vi "Vision Processing.vi"(8 "error in (no error)":errorcluster, 11 "Image Size":T2=enum."320x240") -> ()   [LabVIEW 2015]
uses:
  <vilib>/Rock Robotics/WPI/Camera/WPI_CameraImageSize.ctl
  OS6 VIs/References/Relevant Data.ctl
  Robot Global Data.vi
  <vilib>/vision/NI_Vision_Development_Module.lvlib
panel:
  out "Relevant Data":T1[](array[typedef])
  out "Distance":dbl
  in  "Goal Width":dbl=20.0
  in  "Center Right":dbl=162.0
  in  "Center Left":dbl=153.0
  in  "Mask Color":i32=1
  out "ms to process":u32
  in  "LED Color":T3={"Hue"={91.12518353230051, 179.40124989546868}, "Sat"={197.32142857142858, 255.0}, "Val"={182.14285714285714, 255.0}} {"Hue" scale=0.0..255.0 scale format="%#_3g"}
  out "Qualified Particles":i32
  in  "Aspect Fudge Factor":dbl=1.0
  in  "Min Score Threshold":i32=75
  out "Masked":T4(plugin-control)
  out "Original Image":T4(plugin-control)
  out "fps":dbl
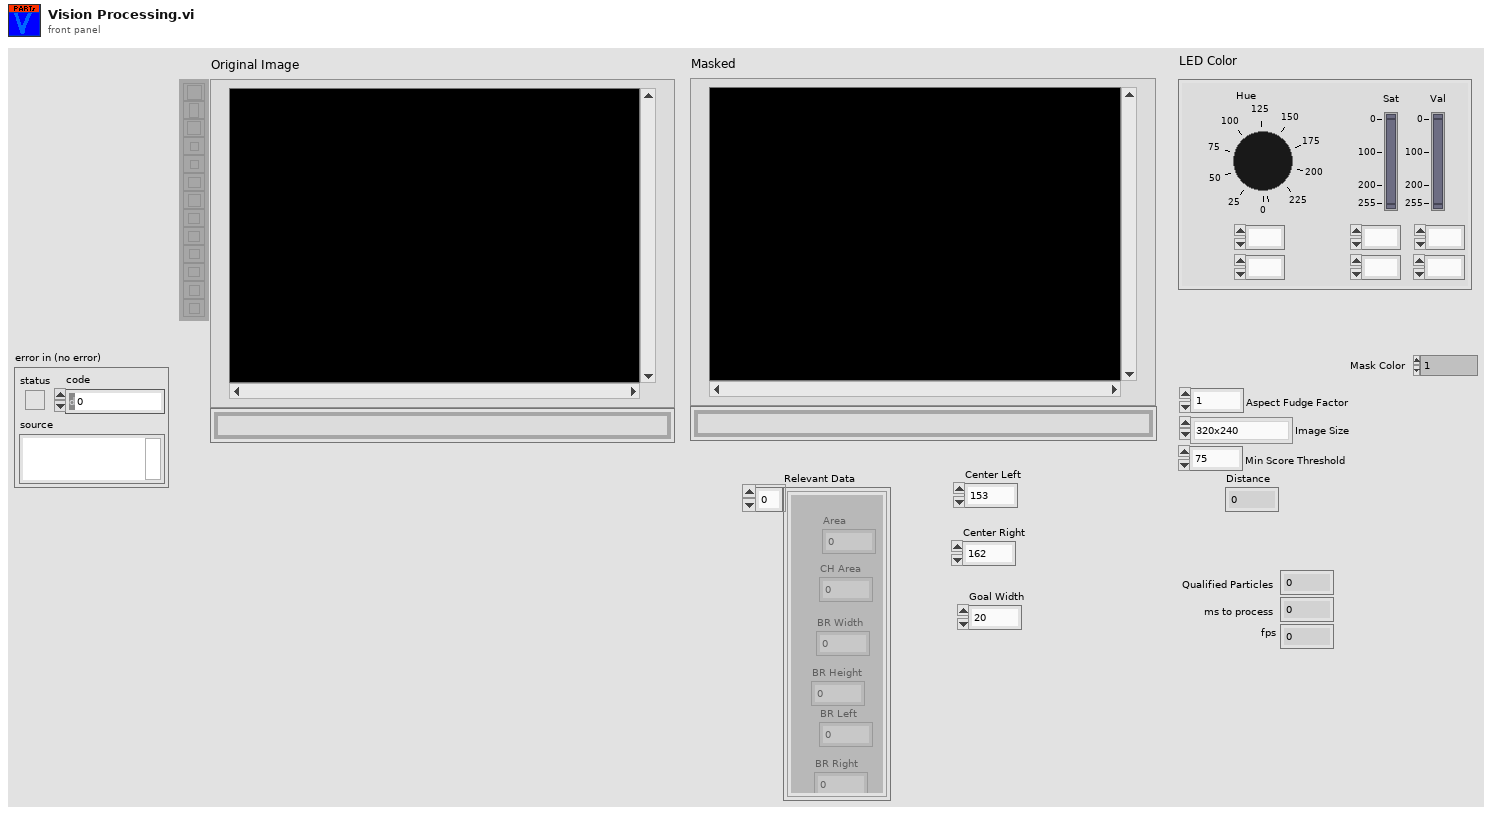
[diagram p1: front panel]
types:
  T1 = typedef "Relevant Data.ctl" = cluster{"Area":dbl, "CH Area":dbl, "BR Width":dbl, "BR Height":dbl, "BR Left":dbl, "BR Right":dbl}
  T2 = typedef "WPI_CameraImageSize.ctl" = enum16{"640x480", "320x240", "160x120", "Custom"}
  T3 = cluster{"Hue":cluster{dbl, dbl}, "Sat":cluster{dbl, dbl}, "Val":cluster{dbl, dbl}}
  T4 = typedef "IMAQ Image.ctl" = refnum<image>
  T5 = typedef "Image Type" = u32
  T6 = typedef "Particle Parameters" = i32
  T7 = typedef "WPI_CameraDevRef.ctl" = cluster{"Camera Address":string, "CameraStatus":errorcluster}
  T8 = cluster{"Goal Left":dbl, "Goal Right":dbl, "Goal Width":dbl}
  T9 = cluster{"Bounding box":cluster{"left":dbl, "top":dbl, "right":dbl, "bottom":dbl}, "Aspect Ratio":dbl, "Area to CH":dbl, "X Mask":dbl, "Y Mask":dbl, "Moment":dbl}[]
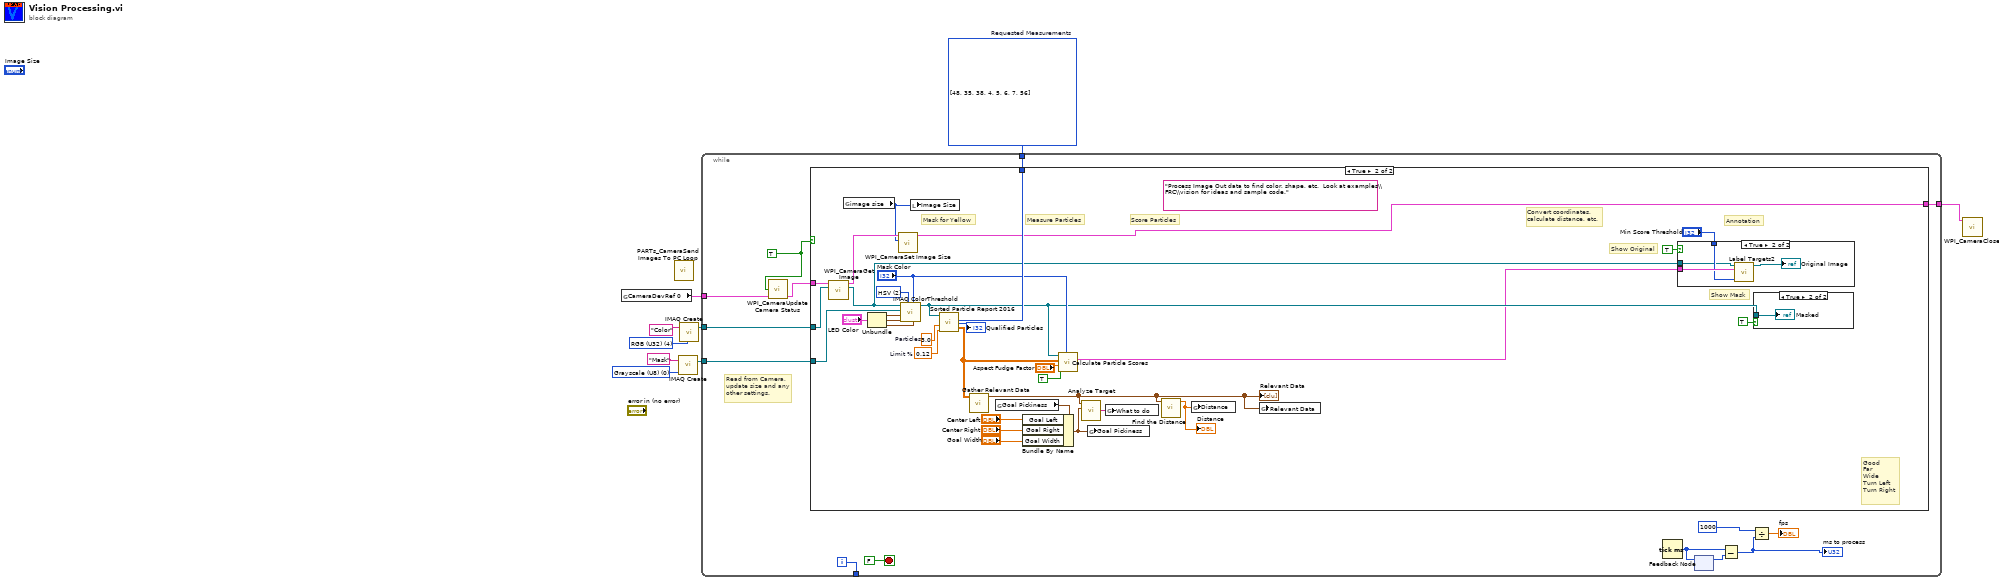
[diagram p0: block diagram]
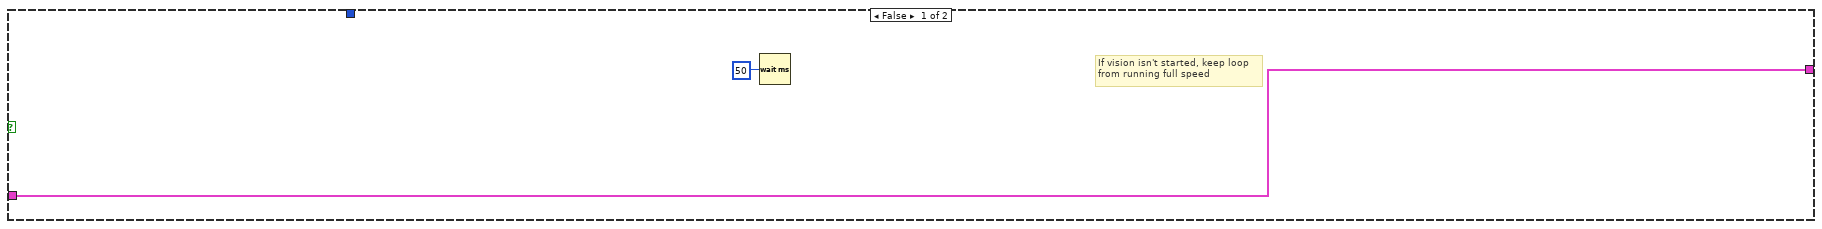
[diagram p2: hidden frame]
diagram:
  w5 = T5 4 items=["Grayscale (U8)", "Grayscale (I16)", "Grayscale (SGL)", "Complex (CSG)", "RGB (U32)", "HSL (U32)", "RGB (U64)", "Grayscale (U16)"] ("Image Type")
  w7 = T6[] [48, 35, 38, 4, 5, 6, 7, 56] items=["Center of Mass X", "Center of Mass Y", "First Pixel X", "First Pixel Y", "Bounding Rect Left", "Bounding Rect Top", "Bounding Rect Right", "Bounding Rect Bottom", "Max Feret Diameter Start X", "Max Feret Diameter Start Y", "Max Feret Diameter End X", "Max Feret Diameter End Y", "Max Horiz. Segment Length Left", "Max Horiz. Segment Length Right", "Max Horiz. Segment Length Row", "-", "Bounding Rect Width", "Bounding Rect Height", "Bounding Rect Diagonal", "Perimeter", "Convex Hull Perimeter", "Holes' Perimeter", "Max Feret Diameter", "Equivalent Ellipse Major Axis", "Equivalent Ellipse Minor Axis", "Equivalent Ellipse Minor Axis (Feret)", "Equivalent Rect Long Side", "Equivalent Rect Short Side", "Equivalent Rect Diagonal", "Equivalent Rect Short Side (Feret)", "Average Horiz. Segment Length", "Average Vert. Segment Length", "Hydraulic Radius", "Waddel Disk Diameter", "-", "Area", "Holes' Area", "Particle & Holes' Area", "Convex Hull Area", "Image Area", "-", "Number of Holes", "Number of Horiz. Segments", "Number of Vert. Segments", "-", "Orientation", "Max Feret Diameter Orientation", "-", "% Area/Image Area", "% Area/(Particle & Holes' Area)", "Ratio of Equivalent Ellipse Axes", "Ratio of Equivalent Rect Sides", "-", "Elongation Factor", "Compactness Factor", "Heywood Circularity Factor", "Type Factor", "-", "Sum X", "Sum Y", "Sum XX", "Sum XY", "Sum YY", "Sum XXX", "Sum XXY", "Sum XYY", "Sum YYY", "-", "Moment of Inertia XX", "Moment of Inertia XY", "Moment of Inertia YY", "Moment of Inertia XXX", "Moment of Inertia XXY", "Moment of Inertia XYY", "Moment of Inertia YYY", "Norm. Moment of Inertia XX", "Norm. Moment of Inertia XY", "Norm. Moment of Inertia YY", "Norm. Moment of Inertia XXX", "Norm. Moment of Inertia XXY", "Norm. Moment of Inertia XYY", "Norm. Moment of Inertia YYY", "Hu Moment 1", "Hu Moment 2", "Hu Moment 3", "Hu Moment 4", "Hu Moment 5", "Hu Moment 6", "Hu Moment 7"]  # Requested Measurements
  w9 = T5 0 items=["Grayscale (U8)", "Grayscale (I16)", "Grayscale (SGL)", "Complex (CSG)", "RGB (U32)", "HSL (U32)", "RGB (U64)", "Grayscale (U16)"] ("Image Type")
  n1 = global read "Robot Global Data.vi" "CameraDevRef 0"() -> (w1:T7)
  n2 = call "PARTs_CameraSend Images To PC Loop.vi"() -> ()  [unwired: 12 in]
  n3 = call "IMAQ Create"("Image Name"="Mask", "Image Type"=w9) -> ("New Image"=w8:T4)  [unwired: 2 in, 2 out]
  n4 = call "IMAQ Create"("Image Name"="Color", "Image Type"=w5) -> ("New Image"=w4:T4)  [unwired: 3 in, 1 out]
  n5 = while {
    tunnel: w8 -> [w22]
    tunnel: w7 -> [w21]
    tunnel: [w18] -> _
    tunnel: w4 -> [w15]
    tunnel: [w13] -> w2
    tunnel: w1 -> [w11]
    i -> [w18]
    stop <- FALSE stop-if-true
    w10 = TRUE
    # "Read from Camera,\nupdate size and any\nother settings."
    n6 = call <vilib>:"WPI_CameraUpdate Camera Status.vi"("CameraDevRef In"=w11, "Enable Vision"=w10) -> ("CameraDevRef Out"=w14:T7)  [unwired: 3 in]
    n7 = case shown="True" w10 {
      tunnel: w22 -> [_ w58]
      tunnel: w21 -> [_ w51]
      tunnel: w15 -> [_ w42]
      tunnel: w14 -> [w24 w43]
      tunnel: [w24 w39] -> w13
      frame False {
        # "If vision isn't started, keep loop\nfrom running full speed"
        n8 = Wait (ms)(milliseconds to wait=u32 50) -> ()  [unwired: 1 out]
      }
      frame True {
        w53 = u16 2 items=["RGB", "HSL", "HSV", "HSI"] ("Color Mode")
        (unwired) "Process Image Out data to find color, shape, etc.  Look at examples\\FRC\\vision for ideas and sample code."
        w50 = 0.12  # Limit %
        w49 = 3.0  # Particles
        # "Show Mask"
        # "Show Original"
        # "Good\nFar\nWide\nTurn Left\nTurn Right"
        # "Measure Particles"
        # "Convert coordinates,\ncalculate distance, etc."
        # "Annotation"
        # "Score Particles"
        # "Mask for Yellow"
        n9 = call <vilib>:"WPI_CameraGet Image.vi"("Image"=w42, "CameraDevRef"=w43) -> ("Image Out"=w37:T4, "CameraDevRef Out"=w41:T7)  [unwired: 7 in, 1 out]
        n10 = global read "Robot Global Data.vi" "image size"() -> (w40:T2)
        n11 = Unbundle("LED Color") -> ("Hue"=w57:cluster{dbl, dbl}, "Sat"=w56:cluster{dbl, dbl}, "Val"=w55:cluster{dbl, dbl})
        n12 = call <vilib>:"WPI_CameraSet Image Size.vi"("Image Size"=w40, "CameraDevRef"=w41) -> ("CameraDevRef Out"=w39:T7)  [unwired: 2 in, 7 out]
        n13 = call "IMAQ ColorThreshold"("Blue or Luma or Val or Inten Range"=w55, "Replace Value"="Mask Color", "Green or Sat Range"=w56, "Color Mode"=w53, "Red or Hue Range"=w57, "Image Dst"=w58, "Image Src"=w37) -> ("Image Dst Out"=w30:T4)  [unwired: 3 in, 1 out]
        n14 = local write "Image Size"(w40) -> ()
        n15 = call "Sorted Particle Report 2016.vi"("Min Area Size %"=w50, "Particle Count Limit"=w49, "Pixel Measurements"=w51, "Image in"=w30) -> ("Sorted Data"=w46:dbl[][], "Particles"=→"Qualified Particles":i32)
        n16 = call "Gather Relevant Data.vi"("Sorted Data"=w46) -> ("Array"=w26:T1[])  [unwired: 10 in]
        "Relevant Data" <- w26
        n17 = global read "Robot Global Data.vi" "Goal Pickiness"() -> (w32:T8)
        n18 = Bundle By Name(cluster=w32, "Goal Left"="Center Left", "Goal Right"="Center Right", "Goal Width"="Goal Width") -> (w31:T8)
        n19 = call "Calculate Particle Scores.vi"("Pixel Value"="Mask Color", "Limit Tests?"=TRUE, "Aspect Fudge Factor"="Aspect Fudge Factor", "Sorted Data"=w46, "Image in"=w30) -> ("Scores"=w29:T9)  [unwired: 6 in]
        n20 = call "Analyze Target.vi"("Goal Pickiness"=w31, "Relevant Data"=w26) -> ("What to do"=w38:string)  [unwired: 9 in]
        n21 = global write "Robot Global Data.vi" "Goal Pickiness"(w31) -> ()
        n22 = global write "Robot Global Data.vi" "What to do"(w38) -> ()
        n23 = call "Find the Distance.vi"("Relevant Data"=w26) -> ("Distance"=w36:dbl)  [unwired: 10 in]
        "Distance" <- w36
        n24 = global write "Robot Global Data.vi" "Distance"(w36) -> ()
        n25 = global write "Robot Global Data.vi" "Relevant Data"(w26) -> ()
        n26 = case shown="True" TRUE {
          tunnel: w29 -> [_ w61]
          tunnel: "Min Score Threshold" -> [_ w60]
          tunnel: w37 -> [_ w59]
          frame False {
          }
          frame True {
            n27 = call "Label Targets2.vi"("Score Threshold"=w60, "Targets"=w61, "Image in"=w59) -> ("Image out"=→"Original Image":T4)  [unwired: 8 in]
          }
        }
        n28 = case shown="True" TRUE {
          tunnel: w30 -> [_ w63]
          frame False {
          }
          frame True {
            "Masked" <- w63
          }
        }
      }
    }
    n29 = Tick Count (ms)() -> (millisecond timer value=w19:u32)
    n30 = feedback-in #1(w19) -> ()
    n31 = feedback #1() -> (w20:u32)  [unwired: 1 in]
    n32 = Subtract(x=w19, y=w20) -> (x-y=w12:u32)
    "ms to process" <- w12
    n33 = Divide(x=1000 ("Brightness"), y=w12) -> (x/y=→"fps":dbl)
  }
  n34 = call <vilib>:"WPI_CameraClose.vi"("CameraDevRef"=w2) -> ()  [unwired: 1 in, 10 out]
